vi "setup_MFLI.vi"(1 "Handle In":T1 {"Handle" format="0x%08x"; "Conn" format="0x%08x"}) -> (0 "Handle Out":T1 {"Handle" format="0x%08x"; "Conn" format="0x%08x"})   [LabVIEW 2019]
uses:
  Monitor Communication/zurich_lock_in/MFLIMonitor-Settings-Cluster.ctl
  Equipment/Zurich Instruments LabOne/Public/ziTypeHandle.ctl
  Instrument_Setup.vi
  Equipment/Zurich Instruments LabOne/Public/Configure/ziSetValueDouble.vi
  Equipment/Zurich Instruments LabOne/Zurich Instruments LabOne.lvlib
panel:
  out "MFLI-1-Settings":T2={"Adress"="DEV4756", "Osc 0 Freq"=0.0, "Osc 1 Freq"=0.0, "Osc 2 Freq"=0.0, "Osc 3 Freq"=0.0, "Demod 0 Osc"=0, "Demod 0 Harm"=1, "Demod 0 Phase"=0.0, "Demod 1 Osc"=0, "Demod 2 Osc"=0, "Demod 3 Osc"=0, "Demod 1 Harm"=1, "Demod 2 Harm"=1, "Demod 3 Harm"=1, "Demod 1 Phase"=0.0, "Demod 2 Phase"=0.0, "Demod 3 Phase"=0.0, "Input Demod 0"="", "Input Demod 1"="", "Input Demod 2"="", "Input Demod 3"="", "Demod 0 Order"=1, "Demod 0 TC"=0.0, "Demod 0 Sinc"=FALSE, "Demod 1 Order"=1, "Demod 2 Order"=1, "Demod 3 Order"=1, "Demod 1 TC"=0.0, "Demod 2 TC"=0.0, "Demod 3 TC"=0.0, "Demod 1 Sinc"=FALSE, "Demod 2 Sinc"=FALSE, "Demod 3 Sinc"=FALSE, "Demod 0 Enable"=FALSE, "Demod 0 Data Rate"=0.0, "Demod 1 Enable"=FALSE, "Demod 2 Enable"=FALSE, "Demod 3 Enable"=FALSE, "Demod 1 Data Rate"=0.0, "Demod 2 Data Rate"=0.0, "Demod 3 Data Rate"=0.0, "Ampl 0"=0.0, "Ampl 0 Enable"=FALSE, "Ampl 1"=0.0, "Ampl 2"=0.0, "Ampl 3"=0.0, "Ampl 1 Enable"=FALSE, "Ampl 2 Enable"=FALSE, "Ampl 3 Enable"=FALSE, "On"=FALSE, "50 Ohm"=FALSE, "Range (V)"=0.0, "Add"=FALSE, "Diff"=FALSE, "Auto-Range"=FALSE, "Offset (V)"=0.0, "Aux Out 0 Select"="", "Aux Out 0 Demod Num"=0.0, "Aux Out 0 Pre Offset"=0.0, "Aux Out 0 Scale"=0.0, "Aux Out 0 Offset"=0.0, "Aux Out 1 Select"="", "Aux Out 2 Select"="", "Aux Out 3 Select"="", "Aux Out 1 Pre Offset"=0.0, "Aux Out 2 Pre Offset"=0.0, "Aux Out 3 Pre Offset"=0.0, "Aux Out 1 Scale"=0.0, "Aux Out 2 Scale"=0.0, "Aux Out 3 Scale"=0.0, "Aux Out 1 Offset"=0.0, "Aux Out 2 Offset"=0.0, "Aux Out 3 Offset"=0.0, "Aux Out 1 Demod Num"=0.0, "Aux Out 2 Demod Num "=0.0, "Aux Out 3 Demod Num"=0.0, "Output Range (V)"=0.0} {"Aux Out 3 Demod Num" min=0.0 max=3.0 step=1.0; "Aux Out 2 Demod Num" min=0.0 max=3.0 step=1.0; "Aux Out 1 Demod Num" min=0.0 max=3.0 step=1.0; "Aux Out 0 Demod Num" min=0.0 max=3.0 step=1.0; "Demod 3 TC" min=0.0; "Demod 2 TC" min=0.0; "Demod 1 TC" min=0.0; "Demod 3 Order" min=1 max=8 step=1; "Demod 2 Order" min=1 max=8 step=1; "Demod 1 Order" min=1 max=8 step=1; "Demod 0 TC" min=0.0; "Demod 0 Order" min=1 max=8 step=1; "Demod 3 Phase" min=0.0 max=360.0; "Demod 2 Phase" min=0.0 max=360.0; "Demod 1 Phase" min=0.0 max=360.0; "Demod 3 Harm" min=1 max=1023 step=1; "Demod 2 Harm" min=1 max=1023 step=1; "Demod 1 Harm" min=1 max=1023 step=1; "Demod 3 Osc" min=0 max=3 step=1; "Demod 2 Osc" min=0 max=3 step=1; "Demod 1 Osc" min=0 max=3 step=1; "Demod 0 Phase" min=0.0 max=360.0; "Demod 0 Harm" min=1 max=1023 step=1; "Demod 0 Osc" min=0 max=3 step=1; "Osc 3 Freq" min=0.0 max=510000.0 format="%#_11g"; "Osc 2 Freq" min=0.0 max=510000.0 format="%#_11g"; "Osc 1 Freq" min=0.0 max=510000.0 format="%#_11g"; "Osc 0 Freq" min=0.0 max=510000.0 format="%#_11g"}
  # "Oscillators"
  # "Demodulators"
  # "Low-Pass Filter"
  # "Data Transfer"
  # "Output Amplitudes"
  # "Signal Outputs"
  # "Frequency (Hz)"
  # "Osc (#)"
  # "Harm (#)"
  # "Phase Offset (°)"
  # "Input"
  # "Order (#)"
  # "TC (s)"
  # "Sinc"
  # "Enabled"
  # "Rate (1/s)"
  # "Ampl (Vpk)"
  # "Enable"
  # "0"
  # "0"
  # "0"
  # "1"
  # "1"
  # "1"
  # "2"
  # "2"
  # "2"
  # "3"
  # "3"
  # "3"
  # "Output"
  # "Demod"
  # "Pre Offset"
  # "Scale"
  # "Offset"
  # "0"
  # "1"
  # "2"
  # "3"
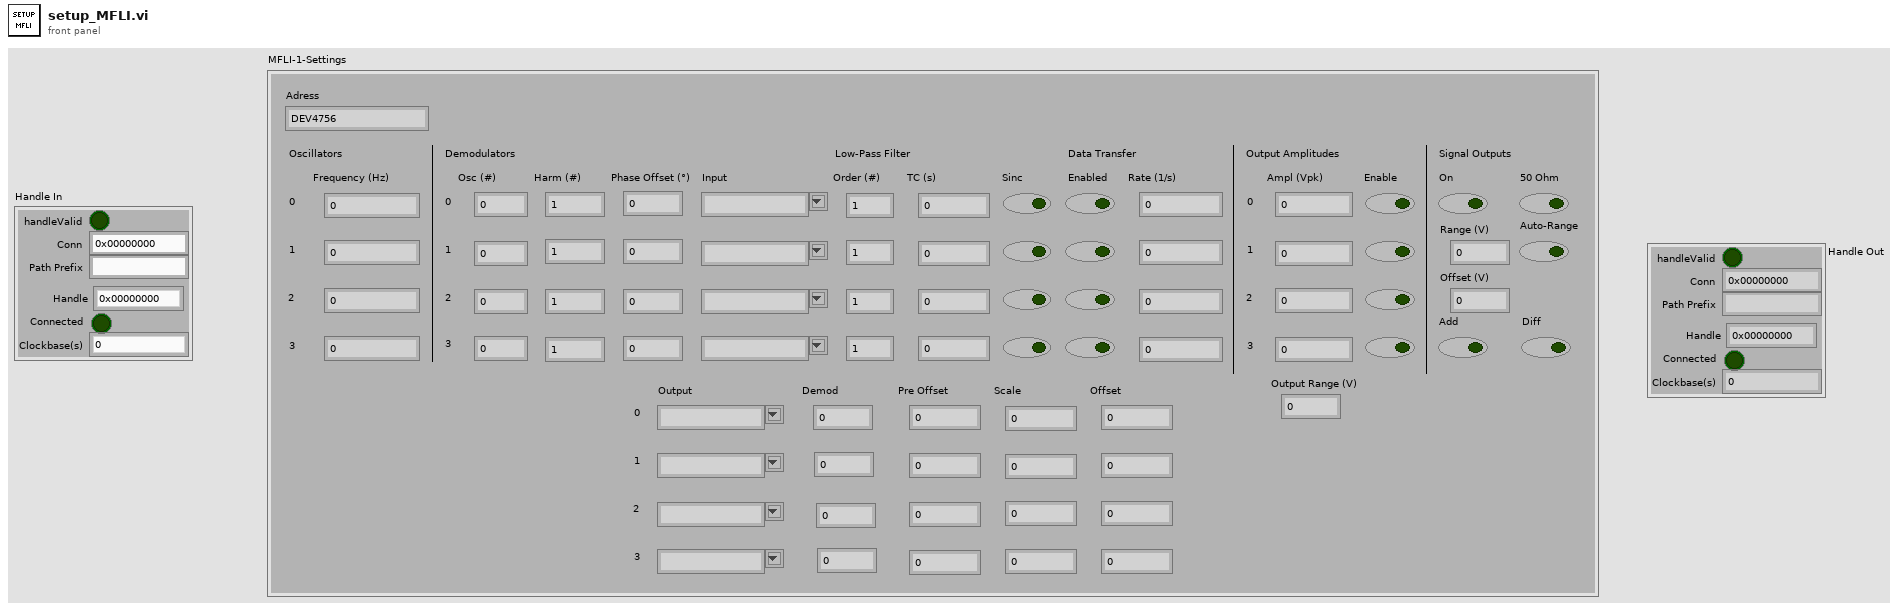
[diagram p1: front panel]
types:
  T1 = typedef "Zurich Instruments LabOne.lvlib/ziTypeHandle.ctl" = cluster{"handleValid":bool, "Conn":u64, "Path Prefix":string, "Handle":u64, "Connected":bool, "Clockbase(s)":dbl}
  T2 = typedef "MFLIMonitor-Settings-Cluster.ctl" = cluster{"Adress":string, "Osc 0 Freq":dbl, "Osc 1 Freq":dbl, "Osc 2 Freq":dbl, "Osc 3 Freq":dbl, "Demod 0 Osc":i8, "Demod 0 Harm":i16, "Demod 0 Phase":dbl, "Demod 1 Osc":i8, "Demod 2 Osc":i8, "Demod 3 Osc":i8, "Demod 1 Harm":i16, "Demod 2 Harm":i16, "Demod 3 Harm":i16, "Demod 1 Phase":dbl, "Demod 2 Phase":dbl, "Demod 3 Phase":dbl, "Input Demod 0":string, "Input Demod 1":string, "Input Demod 2":string, "Input Demod 3":string, "Demod 0 Order":i8, "Demod 0 TC":dbl, "Demod 0 Sinc":bool, "Demod 1 Order":i8, "Demod 2 Order":i8, "Demod 3 Order":i8, "Demod 1 TC":dbl, "Demod 2 TC":dbl, "Demod 3 TC":dbl, "Demod 1 Sinc":bool, "Demod 2 Sinc":bool, "Demod 3 Sinc":bool, "Demod 0 Enable":bool, "Demod 0 Data Rate":dbl, "Demod 1 Enable":bool, "Demod 2 Enable":bool, "Demod 3 Enable":bool, "Demod 1 Data Rate":dbl, "Demod 2 Data Rate":dbl, "Demod 3 Data Rate":dbl, "Ampl 0":dbl, "Ampl 0 Enable":bool, "Ampl 1":dbl, "Ampl 2":dbl, "Ampl 3":dbl, "Ampl 1 Enable":bool, "Ampl 2 Enable":bool, "Ampl 3 Enable":bool, "On":bool, "50 Ohm":bool, "Range (V)":dbl, "Add":bool, "Diff":bool, "Auto-Range":bool, "Offset (V)":dbl, "Aux Out 0 Select":string, "Aux Out 0 Demod Num":dbl, "Aux Out 0 Pre Offset":dbl, "Aux Out 0 Scale":dbl, "Aux Out 0 Offset":dbl, "Aux Out 1 Select":string, "Aux Out 2 Select":string, "Aux Out 3 Select":string, "Aux Out 1 Pre Offset":dbl, "Aux Out 2 Pre Offset":dbl, "Aux Out 3 Pre Offset":dbl, "Aux Out 1 Scale":dbl, "Aux Out 2 Scale":dbl, "Aux Out 3 Scale":dbl, "Aux Out 1 Offset":dbl, "Aux Out 2 Offset":dbl, "Aux Out 3 Offset":dbl, "Aux Out 1 Demod Num":dbl, "Aux Out 2 Demod Num ":dbl, "Aux Out 3 Demod Num":dbl, "Output Range (V)":dbl}
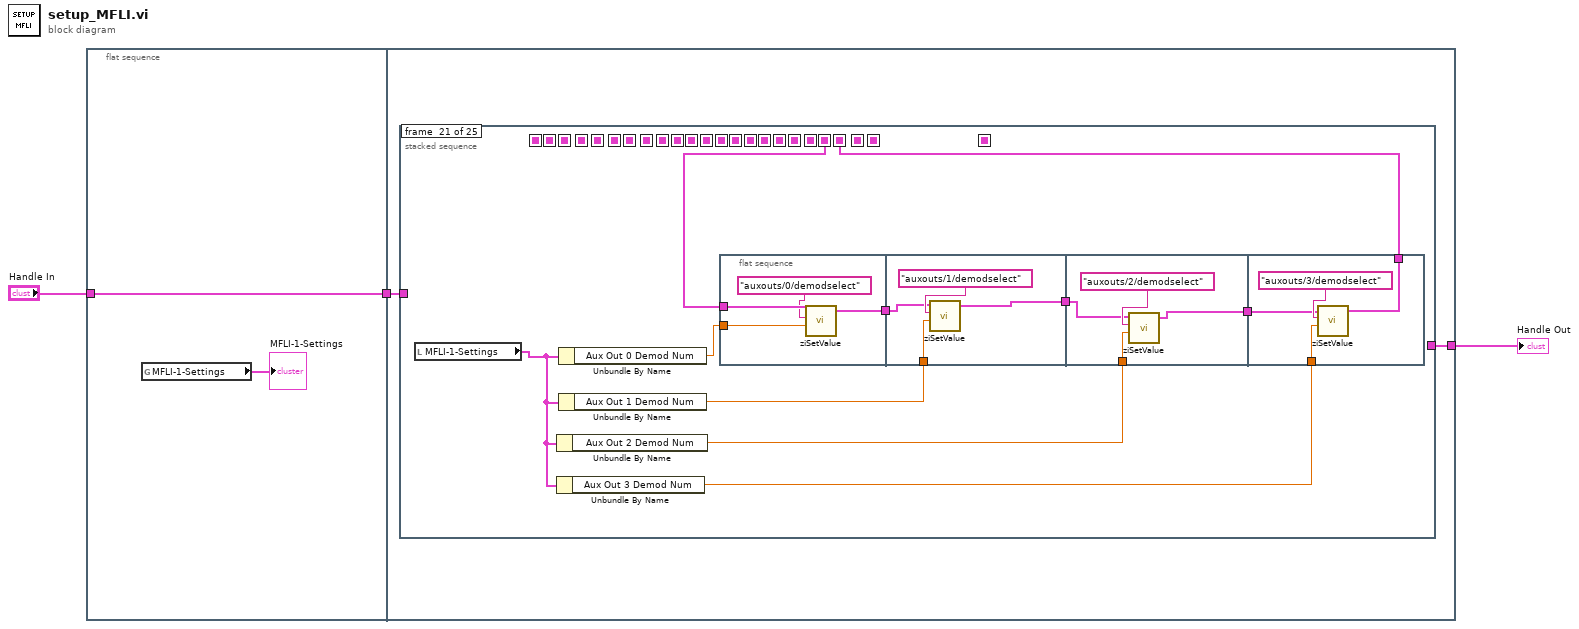
[diagram p0: block diagram]
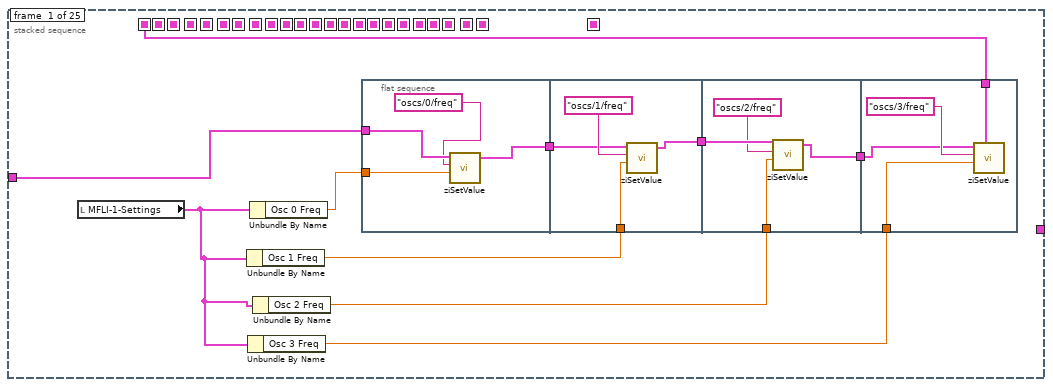
[diagram p2: hidden frame]
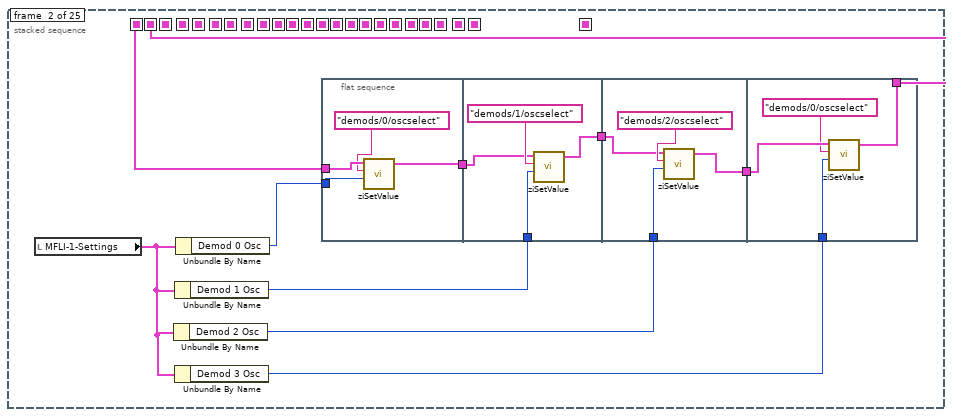
[diagram p3: hidden frame]
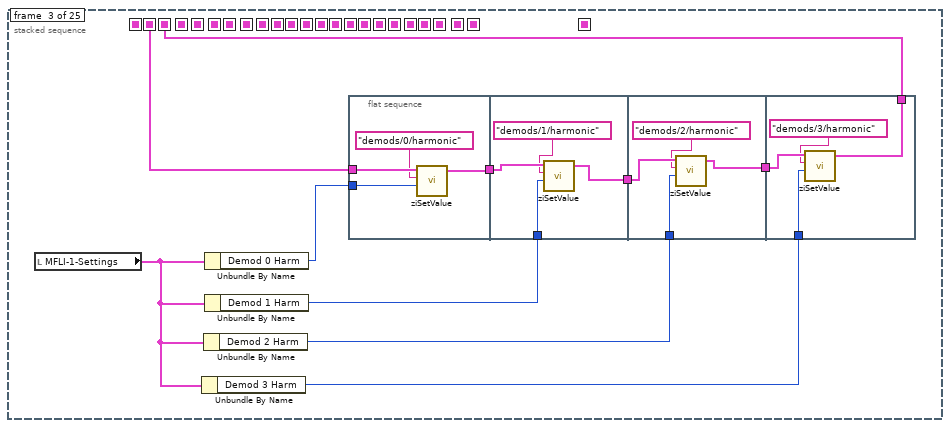
[diagram p4: hidden frame]
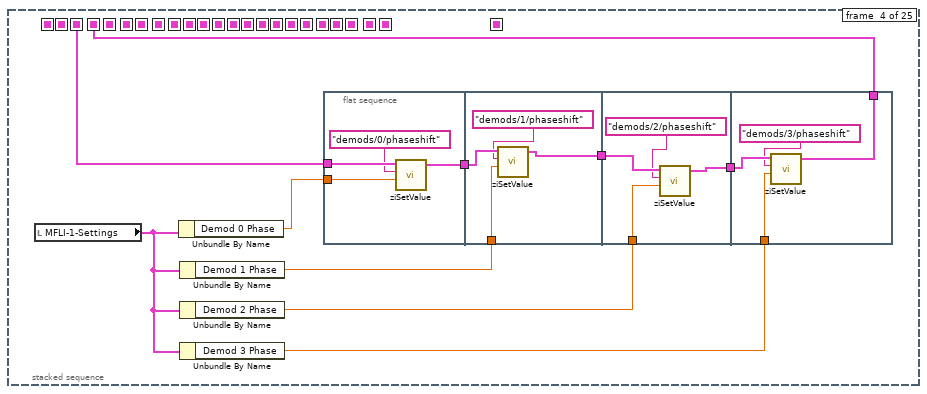
[diagram p5: hidden frame]
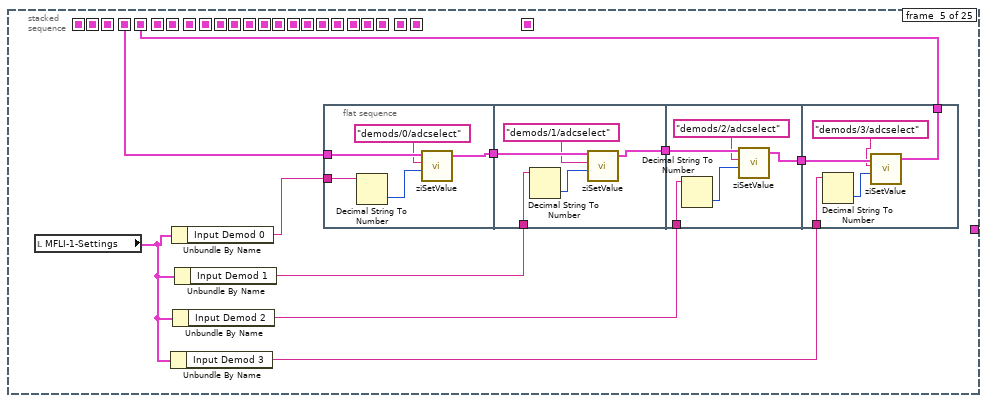
[diagram p6: hidden frame]
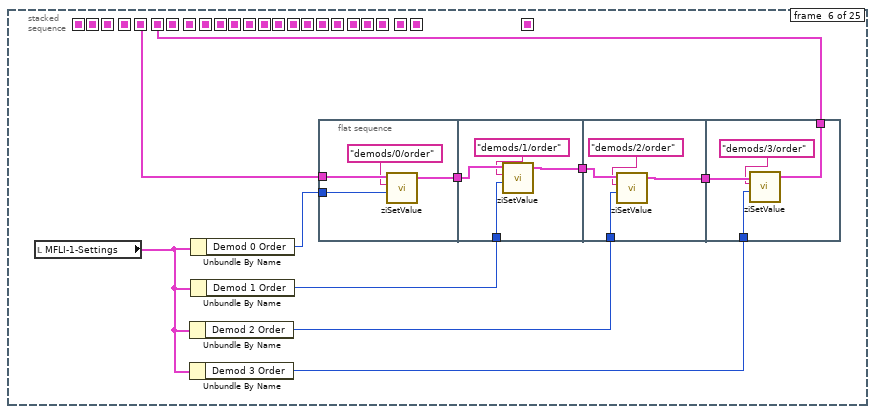
[diagram p7: hidden frame]
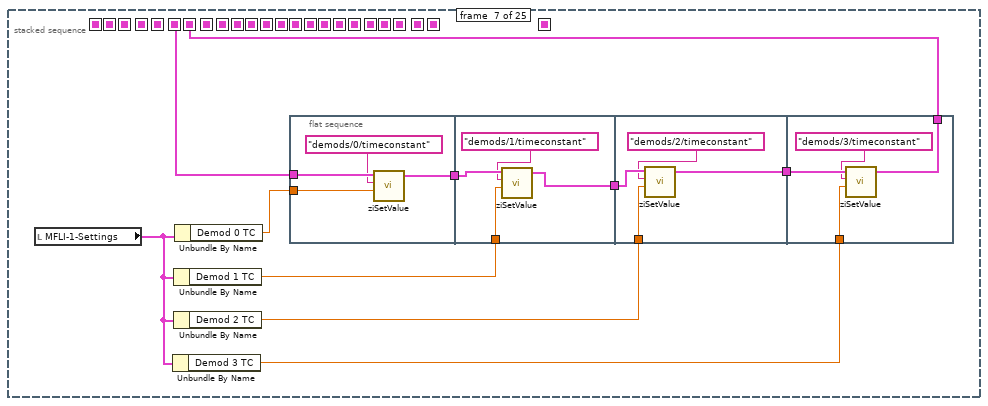
[diagram p8: hidden frame]
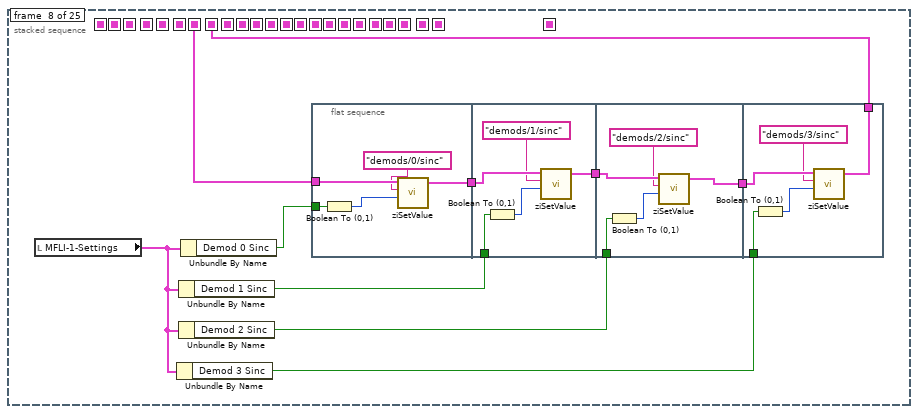
[diagram p9: hidden frame]
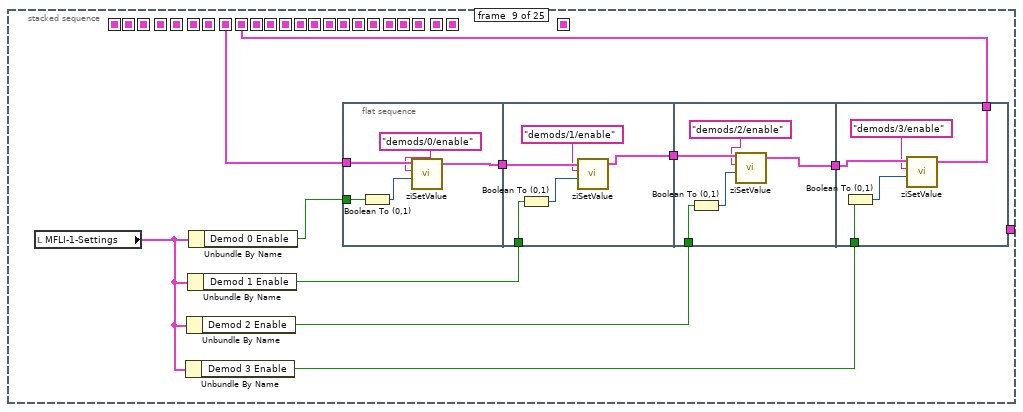
[diagram p10: hidden frame]
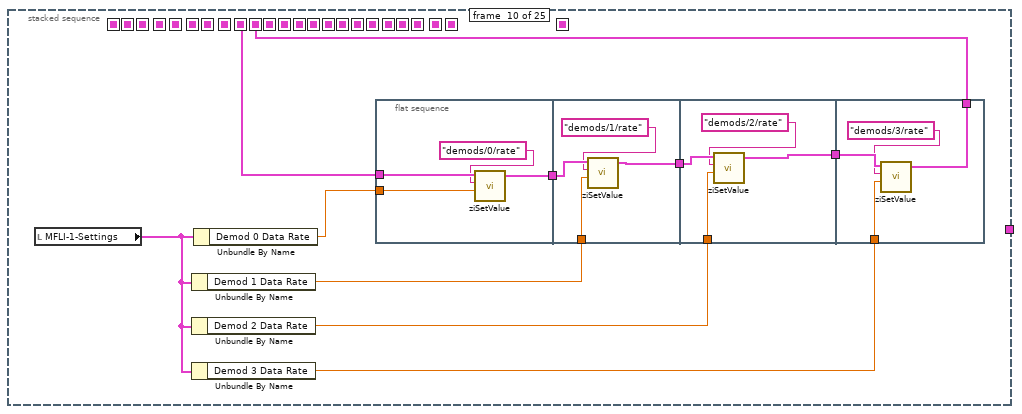
[diagram p11: hidden frame]
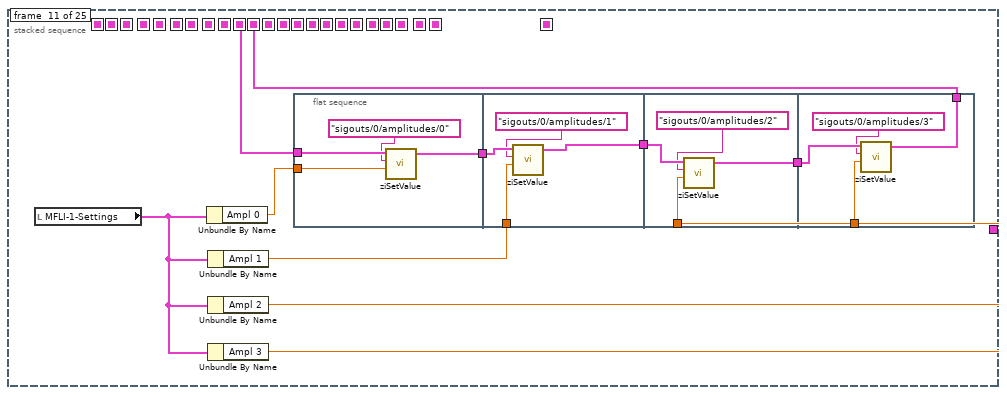
[diagram p12: hidden frame]
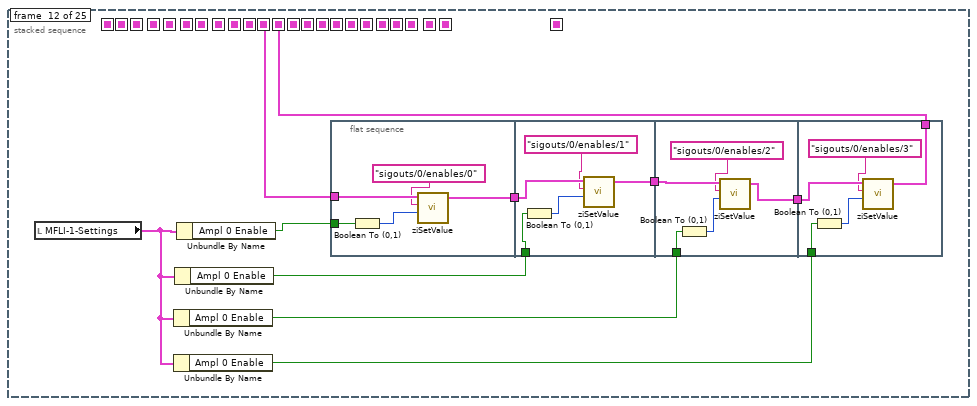
[diagram p13: hidden frame]
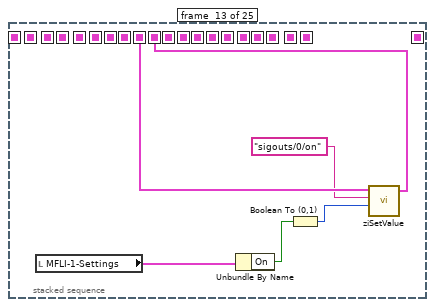
[diagram p14: hidden frame]
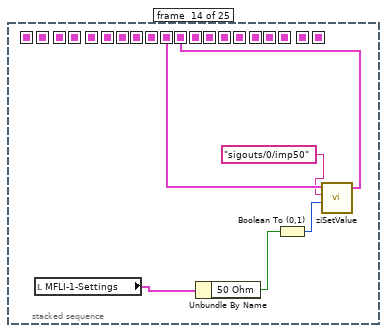
[diagram p15: hidden frame]
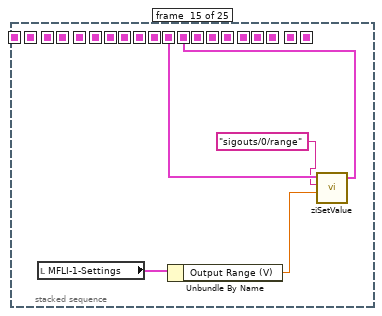
[diagram p16: hidden frame]
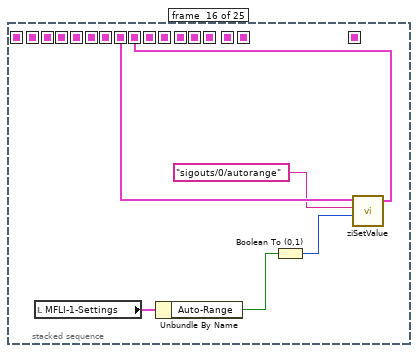
[diagram p17: hidden frame]
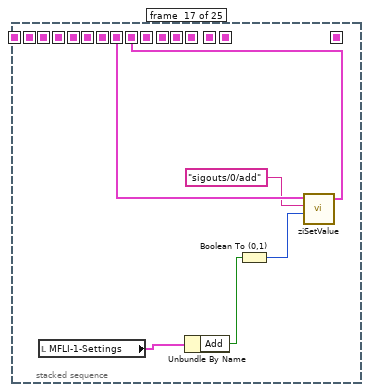
[diagram p18: hidden frame]
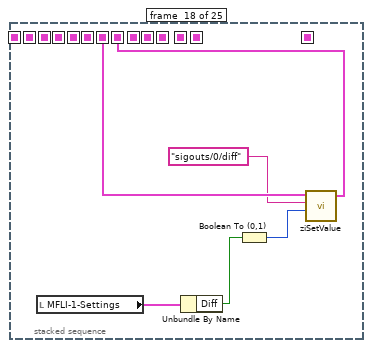
[diagram p19: hidden frame]
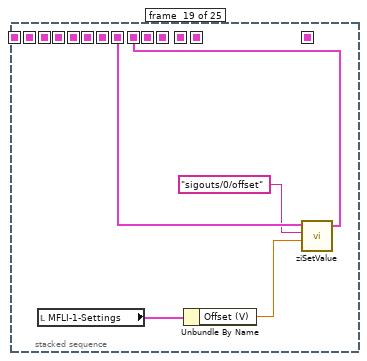
[diagram p20: hidden frame]
diagram:
  n1 = flat-sequence {
    tunnel: "Handle In" -> [w5]
    tunnel: [w5] -> w1
    tunnel: [w6] -> w2
    tunnel: w1 -> [w7]
    frame #0 {
      n2 = global read "Instrument_Setup.vi" "MFLI-1-Settings"() -> (→"MFLI-1-Settings":T2)
    }
    frame #1 {
      n3 = stacked-sequence {
        seq-local: [w8 _ _ _ _ _ _ _ _ _ _ _ _ _ _ _ _ _ _ _ _ _ _ _ _] -> [_ w43 _ _ _ _ _ _ _ _ _ _ _ _ _ _ _ _ _ _ _ _ _ _ _]
        seq-local: [_ w34 _ _ _ _ _ _ _ _ _ _ _ _ _ _ _ _ _ _ _ _ _ _ _] -> [_ _ w69 _ _ _ _ _ _ _ _ _ _ _ _ _ _ _ _ _ _ _ _ _ _]
        seq-local: [_ _ w60 _ _ _ _ _ _ _ _ _ _ _ _ _ _ _ _ _ _ _ _ _ _] -> [_ _ _ w95 _ _ _ _ _ _ _ _ _ _ _ _ _ _ _ _ _ _ _ _ _]
        seq-local: [_ _ _ w86 _ _ _ _ _ _ _ _ _ _ _ _ _ _ _ _ _ _ _ _ _] -> [_ _ _ _ w121 _ _ _ _ _ _ _ _ _ _ _ _ _ _ _ _ _ _ _ _]
        seq-local: [_ _ _ _ w112 _ _ _ _ _ _ _ _ _ _ _ _ _ _ _ _ _ _ _ _] -> [_ _ _ _ _ w151 _ _ _ _ _ _ _ _ _ _ _ _ _ _ _ _ _ _ _]
        seq-local: [_ _ _ _ _ w142 _ _ _ _ _ _ _ _ _ _ _ _ _ _ _ _ _ _ _] -> [_ _ _ _ _ _ w177 _ _ _ _ _ _ _ _ _ _ _ _ _ _ _ _ _ _]
        seq-local: [_ _ _ _ _ _ w168 _ _ _ _ _ _ _ _ _ _ _ _ _ _ _ _ _ _] -> [_ _ _ _ _ _ _ w203 _ _ _ _ _ _ _ _ _ _ _ _ _ _ _ _ _]
        seq-local: [_ _ _ _ _ _ _ w194 _ _ _ _ _ _ _ _ _ _ _ _ _ _ _ _ _] -> [_ _ _ _ _ _ _ _ w233 _ _ _ _ _ _ _ _ _ _ _ _ _ _ _ _]
        seq-local: [_ _ _ _ _ _ _ _ w224 _ _ _ _ _ _ _ _ _ _ _ _ _ _ _ _] -> [_ _ _ _ _ _ _ _ _ w263 _ _ _ _ _ _ _ _ _ _ _ _ _ _ _]
        seq-local: [_ _ _ _ _ _ _ _ _ w254 _ _ _ _ _ _ _ _ _ _ _ _ _ _ _] -> [_ _ _ _ _ _ _ _ _ _ w289 _ _ _ _ _ _ _ _ _ _ _ _ _ _]
        seq-local: [_ _ _ _ _ _ _ _ _ _ w280 _ _ _ _ _ _ _ _ _ _ _ _ _ _] -> [_ _ _ _ _ _ _ _ _ _ _ w315 _ _ _ _ _ _ _ _ _ _ _ _ _]
        seq-local: [_ _ _ _ _ _ _ _ _ _ _ w306 _ _ _ _ _ _ _ _ _ _ _ _ _] -> [_ _ _ _ _ _ _ _ _ _ _ _ w341 _ _ _ _ _ _ _ _ _ _ _ _]
        seq-local: [_ _ _ _ _ _ _ _ _ _ _ _ w339 _ _ _ _ _ _ _ _ _ _ _ _] -> [_ _ _ _ _ _ _ _ _ _ _ _ _ w347 _ _ _ _ _ _ _ _ _ _ _]
        seq-local: [_ _ _ _ _ _ _ _ _ _ _ _ _ w345 _ _ _ _ _ _ _ _ _ _ _] -> [_ _ _ _ _ _ _ _ _ _ _ _ _ _ w352 _ _ _ _ _ _ _ _ _ _]
        seq-local: [_ _ _ _ _ _ _ _ _ _ _ _ _ _ w350 _ _ _ _ _ _ _ _ _ _] -> [_ _ _ _ _ _ _ _ _ _ _ _ _ _ _ w357 _ _ _ _ _ _ _ _ _]
        seq-local: [_ _ _ _ _ _ _ _ _ _ _ _ _ _ _ w356 _ _ _ _ _ _ _ _ _] -> [_ _ _ _ _ _ _ _ _ _ _ _ _ _ _ _ w363 _ _ _ _ _ _ _ _]
        seq-local: [_ _ _ _ _ _ _ _ _ _ _ _ _ _ _ _ w362 _ _ _ _ _ _ _ _] -> [_ _ _ _ _ _ _ _ _ _ _ _ _ _ _ _ _ w370 _ _ _ _ _ _ _]
        seq-local: [_ _ _ _ _ _ _ _ _ _ _ _ _ _ _ _ _ w368 _ _ _ _ _ _ _] -> [_ _ _ _ _ _ _ _ _ _ _ _ _ _ _ _ _ _ w375 _ _ _ _ _ _]
        seq-local: [_ _ _ _ _ _ _ _ _ _ _ _ _ _ _ _ _ _ w373 _ _ _ _ _ _] -> [_ _ _ _ _ _ _ _ _ _ _ _ _ _ _ _ _ _ _ w385 _ _ _ _ _]
        seq-local: [_ _ _ _ _ _ _ _ _ _ _ _ _ _ _ _ _ _ _ w376 _ _ _ _ _] -> [_ _ _ _ _ _ _ _ _ _ _ _ _ _ _ _ _ _ _ _ w415 _ _ _ _]
        seq-local: [_ _ _ _ _ _ _ _ _ _ _ _ _ _ _ _ _ _ _ _ w406 _ _ _ _] -> [_ _ _ _ _ _ _ _ _ _ _ _ _ _ _ _ _ _ _ _ _ w441 _ _ _]
        seq-local: [_ _ _ _ _ _ _ _ _ _ _ _ _ _ _ _ _ _ _ _ _ w432 _ _ _] -> [_ _ _ _ _ _ _ _ _ _ _ _ _ _ _ _ _ _ _ _ _ _ w467 _ _]
        seq-local: [_ _ _ _ _ _ _ _ _ _ _ _ _ _ _ _ _ _ _ _ _ _ w458 _ _] -> [_ _ _ _ _ _ _ _ _ _ _ _ _ _ _ _ _ _ _ _ _ _ _ w493 _]
        seq-local: [_ _ _ _ _ _ _ _ _ _ _ _ _ _ _ _ _ _ _ _ _ _ _ w484 _] -> [_ _ _ _ _ _ _ _ _ _ _ _ _ _ _ _ _ _ _ _ _ _ _ _ w514]
        tunnel: w7 -> [w17 _ _ _ _ _ _ _ _ _ _ _ _ _ _ _ _ _ _ _ _ _ _ _ _]
        tunnel: [_ _ _ _ _ _ _ _ _ _ _ _ _ _ _ _ _ _ _ _ _ _ _ _ w512] -> w6
        frame #0 {
          n4 = local read "MFLI-1-Settings"() -> (w15:T2)
          n5 = Unbundle By Name(w15) -> ("Osc 1 Freq"=w13:dbl)
          n6 = Unbundle By Name(w15) -> ("Osc 3 Freq"=w9:dbl)
          n7 = Unbundle By Name(w15) -> ("Osc 0 Freq"=w16:dbl)
          n8 = Unbundle By Name(w15) -> ("Osc 2 Freq"=w11:dbl)
          n9 = flat-sequence {
            tunnel: w17 -> [w21]
            tunnel: w16 -> [w18]
            tunnel: [w20] -> w14
            tunnel: w14 -> [w23]
            tunnel: w13 -> [w25]
            tunnel: [w22] -> w12
            tunnel: w12 -> [w28]
            tunnel: w11 -> [w29]
            tunnel: [w27] -> w10
            tunnel: w10 -> [w31]
            tunnel: w9 -> [w33]
            tunnel: [w30] -> w8
            frame #0 {
              n10 = call-poly "ziSetValue.vi"("Value"=w18, "Path"="oscs/0/freq", "Handle In"=w21) -> ("Handle Out"=w20:T1)  [unwired: 2 in, 1 out]
            }
            frame #1 {
              n11 = call-poly "ziSetValue.vi"("Value"=w25, "Path"="oscs/1/freq", "Handle In"=w23) -> ("Handle Out"=w22:T1)  [unwired: 2 in, 1 out]
            }
            frame #2 {
              n12 = call-poly "ziSetValue.vi"("Value"=w29, "Path"="oscs/2/freq", "Handle In"=w28) -> ("Handle Out"=w27:T1)  [unwired: 2 in, 1 out]
            }
            frame #3 {
              n13 = call-poly "ziSetValue.vi"("Value"=w33, "Path"="oscs/3/freq", "Handle In"=w31) -> ("Handle Out"=w30:T1)  [unwired: 2 in, 1 out]
            }
          }
        }
        frame #1 {
          n14 = local read "MFLI-1-Settings"() -> (w42:T2)
          n15 = Unbundle By Name(w42) -> ("Demod 2 Osc"=w37:i8)
          n16 = Unbundle By Name(w42) -> ("Demod 1 Osc"=w39:i8)
          n17 = Unbundle By Name(w42) -> ("Demod 3 Osc"=w35:i8)
          n18 = Unbundle By Name(w42) -> ("Demod 0 Osc"=w41:i8)
          n19 = flat-sequence {
            tunnel: w43 -> [w47]
            tunnel: w41 -> [w44]
            tunnel: [w46] -> w40
            tunnel: w40 -> [w49]
            tunnel: w39 -> [w51]
            tunnel: [w48] -> w38
            tunnel: w38 -> [w53]
            tunnel: w37 -> [w55]
            tunnel: [w52] -> w36
            tunnel: w36 -> [w58]
            tunnel: w35 -> [w59]
            tunnel: [w57] -> w34
            frame #0 {
              n20 = call-poly "ziSetValue.vi"("Value"=w44, "Path"="demods/0/oscselect", "Handle In"=w47) -> ("Handle Out"=w46:T1)  [unwired: 2 in, 1 out]
            }
            frame #1 {
              n21 = call-poly "ziSetValue.vi"("Value"=w51, "Path"="demods/1/oscselect", "Handle In"=w49) -> ("Handle Out"=w48:T1)  [unwired: 2 in, 1 out]
            }
            frame #2 {
              n22 = call-poly "ziSetValue.vi"("Value"=w55, "Path"="demods/2/oscselect", "Handle In"=w53) -> ("Handle Out"=w52:T1)  [unwired: 2 in, 1 out]
            }
            frame #3 {
              n23 = call-poly "ziSetValue.vi"("Value"=w59, "Path"="demods/0/oscselect", "Handle In"=w58) -> ("Handle Out"=w57:T1)  [unwired: 2 in, 1 out]
            }
          }
        }
        frame #2 {
          n24 = local read "MFLI-1-Settings"() -> (w68:T2)
          n25 = Unbundle By Name(w68) -> ("Demod 3 Harm"=w61:i16)
          n26 = Unbundle By Name(w68) -> ("Demod 2 Harm"=w63:i16)
          n27 = Unbundle By Name(w68) -> ("Demod 0 Harm"=w67:i16)
          n28 = Unbundle By Name(w68) -> ("Demod 1 Harm"=w65:i16)
          n29 = flat-sequence {
            tunnel: w69 -> [w73]
            tunnel: w67 -> [w70]
            tunnel: [w72] -> w66
            tunnel: w66 -> [w76]
            tunnel: w65 -> [w77]
            tunnel: [w75] -> w64
            tunnel: w64 -> [w80]
            tunnel: w63 -> [w81]
            tunnel: [w79] -> w62
            tunnel: w62 -> [w84]
            tunnel: w61 -> [w85]
            tunnel: [w83] -> w60
            frame #0 {
              n30 = call-poly "ziSetValue.vi"("Value"=w70, "Path"="demods/0/harmonic", "Handle In"=w73) -> ("Handle Out"=w72:T1)  [unwired: 2 in, 1 out]
            }
            frame #1 {
              n31 = call-poly "ziSetValue.vi"("Value"=w77, "Path"="demods/1/harmonic", "Handle In"=w76) -> ("Handle Out"=w75:T1)  [unwired: 2 in, 1 out]
            }
            frame #2 {
              n32 = call-poly "ziSetValue.vi"("Value"=w81, "Path"="demods/2/harmonic", "Handle In"=w80) -> ("Handle Out"=w79:T1)  [unwired: 2 in, 1 out]
            }
            frame #3 {
              n33 = call-poly "ziSetValue.vi"("Value"=w85, "Path"="demods/3/harmonic", "Handle In"=w84) -> ("Handle Out"=w83:T1)  [unwired: 2 in, 1 out]
            }
          }
        }
        frame #3 {
          n34 = local read "MFLI-1-Settings"() -> (w94:T2)
          n35 = Unbundle By Name(w94) -> ("Demod 0 Phase"=w93:dbl)
          n36 = Unbundle By Name(w94) -> ("Demod 1 Phase"=w91:dbl)
          n37 = Unbundle By Name(w94) -> ("Demod 2 Phase"=w89:dbl)
          n38 = Unbundle By Name(w94) -> ("Demod 3 Phase"=w87:dbl)
          n39 = flat-sequence {
            tunnel: w95 -> [w99]
            tunnel: w93 -> [w96]
            tunnel: [w98] -> w92
            tunnel: w92 -> [w102]
            tunnel: w91 -> [w103]
            tunnel: [w101] -> w90
            tunnel: w90 -> [w106]
            tunnel: w89 -> [w107]
            tunnel: [w105] -> w88
            tunnel: w88 -> [w110]
            tunnel: w87 -> [w111]
            tunnel: [w109] -> w86
            frame #0 {
              n40 = call-poly "ziSetValue.vi"("Value"=w96, "Path"="demods/0/phaseshift", "Handle In"=w99) -> ("Handle Out"=w98:T1)  [unwired: 2 in, 1 out]
            }
            frame #1 {
              n41 = call-poly "ziSetValue.vi"("Value"=w103, "Path"="demods/1/phaseshift", "Handle In"=w102) -> ("Handle Out"=w101:T1)  [unwired: 2 in, 1 out]
            }
            frame #2 {
              n42 = call-poly "ziSetValue.vi"("Value"=w107, "Path"="demods/2/phaseshift", "Handle In"=w106) -> ("Handle Out"=w105:T1)  [unwired: 2 in, 1 out]
            }
            frame #3 {
              n43 = call-poly "ziSetValue.vi"("Value"=w111, "Path"="demods/3/phaseshift", "Handle In"=w110) -> ("Handle Out"=w109:T1)  [unwired: 2 in, 1 out]
            }
          }
        }
        frame #4 {
          n44 = local read "MFLI-1-Settings"() -> (w120:T2)
          n45 = Unbundle By Name(w120) -> ("Input Demod 3"=w113:string)
          n46 = Unbundle By Name(w120) -> ("Input Demod 0"=w119:string)
          n47 = Unbundle By Name(w120) -> ("Input Demod 2"=w115:string)
          n48 = Unbundle By Name(w120) -> ("Input Demod 1"=w117:string)
          n49 = flat-sequence {
            tunnel: w121 -> [w126]
            tunnel: w119 -> [w122]
            tunnel: [w125] -> w118
            tunnel: w118 -> [w129]
            tunnel: w117 -> [w131]
            tunnel: [w128] -> w116
            tunnel: w116 -> [w134]
            tunnel: w115 -> [w136]
            tunnel: [w133] -> w114
            tunnel: w114 -> [w139]
            tunnel: w113 -> [w141]
            tunnel: [w138] -> w112
            frame #0 {
              n50 = Decimal String To Number(string=w122) -> (number=w123:i32)  [unwired: 2 in, 1 out]
              n51 = call-poly "ziSetValue.vi"("Value"=w123, "Path"="demods/0/adcselect", "Handle In"=w126) -> ("Handle Out"=w125:T1)  [unwired: 2 in, 1 out]
            }
            frame #1 {
              n52 = Decimal String To Number(string=w131) -> (number=w130:i32)  [unwired: 2 in, 1 out]
              n53 = call-poly "ziSetValue.vi"("Value"=w130, "Path"="demods/1/adcselect", "Handle In"=w129) -> ("Handle Out"=w128:T1)  [unwired: 2 in, 1 out]
            }
            frame #2 {
              n54 = Decimal String To Number(string=w136) -> (number=w135:i32)  [unwired: 2 in, 1 out]
              n55 = call-poly "ziSetValue.vi"("Value"=w135, "Path"="demods/2/adcselect", "Handle In"=w134) -> ("Handle Out"=w133:T1)  [unwired: 2 in, 1 out]
            }
            frame #3 {
              n56 = Decimal String To Number(string=w141) -> (number=w140:i32)  [unwired: 2 in, 1 out]
              n57 = call-poly "ziSetValue.vi"("Value"=w140, "Path"="demods/3/adcselect", "Handle In"=w139) -> ("Handle Out"=w138:T1)  [unwired: 2 in, 1 out]
            }
          }
        }
        frame #5 {
          n58 = local read "MFLI-1-Settings"() -> (w150:T2)
          n59 = Unbundle By Name(w150) -> ("Demod 2 Order"=w145:i8)
          n60 = Unbundle By Name(w150) -> ("Demod 3 Order"=w143:i8)
          n61 = Unbundle By Name(w150) -> ("Demod 0 Order"=w149:i8)
          n62 = Unbundle By Name(w150) -> ("Demod 1 Order"=w147:i8)
          n63 = flat-sequence {
            tunnel: w151 -> [w155]
            tunnel: w149 -> [w152]
            tunnel: [w154] -> w148
            tunnel: w148 -> [w158]
            tunnel: w147 -> [w159]
            tunnel: [w157] -> w146
            tunnel: w146 -> [w162]
            tunnel: w145 -> [w163]
            tunnel: [w161] -> w144
            tunnel: w144 -> [w166]
            tunnel: w143 -> [w167]
            tunnel: [w165] -> w142
            frame #0 {
              n64 = call-poly "ziSetValue.vi"("Value"=w152, "Path"="demods/0/order", "Handle In"=w155) -> ("Handle Out"=w154:T1)  [unwired: 2 in, 1 out]
            }
            frame #1 {
              n65 = call-poly "ziSetValue.vi"("Value"=w159, "Path"="demods/1/order", "Handle In"=w158) -> ("Handle Out"=w157:T1)  [unwired: 2 in, 1 out]
            }
            frame #2 {
              n66 = call-poly "ziSetValue.vi"("Value"=w163, "Path"="demods/2/order", "Handle In"=w162) -> ("Handle Out"=w161:T1)  [unwired: 2 in, 1 out]
            }
            frame #3 {
              n67 = call-poly "ziSetValue.vi"("Value"=w167, "Path"="demods/3/order", "Handle In"=w166) -> ("Handle Out"=w165:T1)  [unwired: 2 in, 1 out]
            }
          }
        }
        frame #6 {
          n68 = local read "MFLI-1-Settings"() -> (w176:T2)
          n69 = Unbundle By Name(w176) -> ("Demod 3 TC"=w169:dbl)
          n70 = Unbundle By Name(w176) -> ("Demod 1 TC"=w173:dbl)
          n71 = Unbundle By Name(w176) -> ("Demod 2 TC"=w171:dbl)
          n72 = Unbundle By Name(w176) -> ("Demod 0 TC"=w175:dbl)
          n73 = flat-sequence {
            tunnel: w177 -> [w181]
            tunnel: w175 -> [w178]
            tunnel: [w180] -> w174
            tunnel: w174 -> [w184]
            tunnel: w173 -> [w185]
            tunnel: [w183] -> w172
            tunnel: w172 -> [w188]
            tunnel: w171 -> [w189]
            tunnel: [w187] -> w170
            tunnel: w170 -> [w192]
            tunnel: w169 -> [w193]
            tunnel: [w191] -> w168
            frame #0 {
              n74 = call-poly "ziSetValue.vi"("Value"=w178, "Path"="demods/0/timeconstant", "Handle In"=w181) -> ("Handle Out"=w180:T1)  [unwired: 2 in, 1 out]
            }
            frame #1 {
              n75 = call-poly "ziSetValue.vi"("Value"=w185, "Path"="demods/1/timeconstant", "Handle In"=w184) -> ("Handle Out"=w183:T1)  [unwired: 2 in, 1 out]
            }
            frame #2 {
              n76 = call-poly "ziSetValue.vi"("Value"=w189, "Path"="demods/2/timeconstant", "Handle In"=w188) -> ("Handle Out"=w187:T1)  [unwired: 2 in, 1 out]
            }
            frame #3 {
              n77 = call-poly "ziSetValue.vi"("Value"=w193, "Path"="demods/3/timeconstant", "Handle In"=w192) -> ("Handle Out"=w191:T1)  [unwired: 2 in, 1 out]
            }
          }
        }
        frame #7 {
          n78 = local read "MFLI-1-Settings"() -> (w202:T2)
          n79 = Unbundle By Name(w202) -> ("Demod 3 Sinc"=w195:bool)
          n80 = Unbundle By Name(w202) -> ("Demod 1 Sinc"=w199:bool)
          n81 = Unbundle By Name(w202) -> ("Demod 2 Sinc"=w197:bool)
          n82 = Unbundle By Name(w202) -> ("Demod 0 Sinc"=w201:bool)
          n83 = flat-sequence {
            tunnel: w203 -> [w208]
            tunnel: w201 -> [w204]
            tunnel: [w207] -> w200
            tunnel: w200 -> [w211]
            tunnel: w199 -> [w213]
            tunnel: [w210] -> w198
            tunnel: w198 -> [w216]
            tunnel: w197 -> [w218]
            tunnel: [w215] -> w196
            tunnel: w196 -> [w221]
            tunnel: w195 -> [w223]
            tunnel: [w220] -> w194
            frame #0 {
              n84 = Boolean To (0,1)(Boolean=w204) -> (0, 1=w205:i16)
              n85 = call-poly "ziSetValue.vi"("Value"=w205, "Path"="demods/0/sinc", "Handle In"=w208) -> ("Handle Out"=w207:T1)  [unwired: 2 in, 1 out]
            }
            frame #1 {
              n86 = Boolean To (0,1)(Boolean=w213) -> (0, 1=w212:i16)
              n87 = call-poly "ziSetValue.vi"("Value"=w212, "Path"="demods/1/sinc", "Handle In"=w211) -> ("Handle Out"=w210:T1)  [unwired: 2 in, 1 out]
            }
            frame #2 {
              n88 = Boolean To (0,1)(Boolean=w218) -> (0, 1=w217:i16)
              n89 = call-poly "ziSetValue.vi"("Value"=w217, "Path"="demods/2/sinc", "Handle In"=w216) -> ("Handle Out"=w215:T1)  [unwired: 2 in, 1 out]
            }
            frame #3 {
              n90 = Boolean To (0,1)(Boolean=w223) -> (0, 1=w222:i16)
              n91 = call-poly "ziSetValue.vi"("Value"=w222, "Path"="demods/3/sinc", "Handle In"=w221) -> ("Handle Out"=w220:T1)  [unwired: 2 in, 1 out]
            }
          }
        }
        frame #8 {
          n92 = local read "MFLI-1-Settings"() -> (w232:T2)
          n93 = Unbundle By Name(w232) -> ("Demod 3 Enable"=w225:bool)
          n94 = Unbundle By Name(w232) -> ("Demod 2 Enable"=w227:bool)
          n95 = Unbundle By Name(w232) -> ("Demod 1 Enable"=w229:bool)
          n96 = Unbundle By Name(w232) -> ("Demod 0 Enable"=w231:bool)
          n97 = flat-sequence {
            tunnel: w233 -> [w238]
            tunnel: w231 -> [w234]
            tunnel: [w237] -> w230
            tunnel: w230 -> [w241]
            tunnel: w229 -> [w243]
            tunnel: [w240] -> w228
            tunnel: w228 -> [w246]
            tunnel: w227 -> [w248]
            tunnel: [w245] -> w226
            tunnel: w226 -> [w251]
            tunnel: w225 -> [w253]
            tunnel: [w250] -> w224
            frame #0 {
              n98 = Boolean To (0,1)(Boolean=w234) -> (0, 1=w235:i16)
              n99 = call-poly "ziSetValue.vi"("Value"=w235, "Path"="demods/0/enable", "Handle In"=w238) -> ("Handle Out"=w237:T1)  [unwired: 2 in, 1 out]
            }
            frame #1 {
              n100 = Boolean To (0,1)(Boolean=w243) -> (0, 1=w242:i16)
              n101 = call-poly "ziSetValue.vi"("Value"=w242, "Path"="demods/1/enable", "Handle In"=w241) -> ("Handle Out"=w240:T1)  [unwired: 2 in, 1 out]
            }
            frame #2 {
              n102 = Boolean To (0,1)(Boolean=w248) -> (0, 1=w247:i16)
              n103 = call-poly "ziSetValue.vi"("Value"=w247, "Path"="demods/2/enable", "Handle In"=w246) -> ("Handle Out"=w245:T1)  [unwired: 2 in, 1 out]
            }
            frame #3 {
              n104 = Boolean To (0,1)(Boolean=w253) -> (0, 1=w252:i16)
              n105 = call-poly "ziSetValue.vi"("Value"=w252, "Path"="demods/3/enable", "Handle In"=w251) -> ("Handle Out"=w250:T1)  [unwired: 2 in, 1 out]
            }
          }
        }
        frame #9 {
          n106 = local read "MFLI-1-Settings"() -> (w262:T2)
          n107 = Unbundle By Name(w262) -> ("Demod 1 Data Rate"=w259:dbl)
          n108 = Unbundle By Name(w262) -> ("Demod 2 Data Rate"=w257:dbl)
          n109 = Unbundle By Name(w262) -> ("Demod 3 Data Rate"=w255:dbl)
          n110 = Unbundle By Name(w262) -> ("Demod 0 Data Rate"=w261:dbl)
          n111 = flat-sequence {
            tunnel: w263 -> [w267]
            tunnel: w261 -> [w264]
            tunnel: [w266] -> w260
            tunnel: w260 -> [w270]
            tunnel: w259 -> [w271]
            tunnel: [w269] -> w258
            tunnel: w258 -> [w274]
            tunnel: w257 -> [w275]
            tunnel: [w273] -> w256
            tunnel: w256 -> [w278]
            tunnel: w255 -> [w279]
            tunnel: [w277] -> w254
            frame #0 {
              n112 = call-poly "ziSetValue.vi"("Value"=w264, "Path"="demods/0/rate", "Handle In"=w267) -> ("Handle Out"=w266:T1)  [unwired: 2 in, 1 out]
            }
            frame #1 {
              n113 = call-poly "ziSetValue.vi"("Value"=w271, "Path"="demods/1/rate", "Handle In"=w270) -> ("Handle Out"=w269:T1)  [unwired: 2 in, 1 out]
            }
            frame #2 {
              n114 = call-poly "ziSetValue.vi"("Value"=w275, "Path"="demods/2/rate", "Handle In"=w274) -> ("Handle Out"=w273:T1)  [unwired: 2 in, 1 out]
            }
            frame #3 {
              n115 = call-poly "ziSetValue.vi"("Value"=w279, "Path"="demods/3/rate", "Handle In"=w278) -> ("Handle Out"=w277:T1)  [unwired: 2 in, 1 out]
            }
          }
        }
        frame #10 {
          n116 = local read "MFLI-1-Settings"() -> (w288:T2)
          n117 = Unbundle By Name(w288) -> ("Ampl 0"=w287:dbl)
          n118 = Unbundle By Name(w288) -> ("Ampl 1"=w285:dbl)
          n119 = Unbundle By Name(w288) -> ("Ampl 2"=w283:dbl)
          n120 = Unbundle By Name(w288) -> ("Ampl 3"=w281:dbl)
          n121 = flat-sequence {
            tunnel: w289 -> [w293]
            tunnel: w287 -> [w290]
            tunnel: [w292] -> w286
            tunnel: w286 -> [w296]
            tunnel: w285 -> [w297]
            tunnel: [w295] -> w284
            tunnel: w284 -> [w300]
            tunnel: w283 -> [w301]
            tunnel: [w299] -> w282
            tunnel: w282 -> [w304]
            tunnel: w281 -> [w305]
            tunnel: [w303] -> w280
            frame #0 {
              n122 = call-poly "ziSetValue.vi"("Value"=w290, "Path"="sigouts/0/amplitudes/0", "Handle In"=w293) -> ("Handle Out"=w292:T1)  [unwired: 2 in, 1 out]
            }
            frame #1 {
              n123 = call-poly "ziSetValue.vi"("Value"=w297, "Path"="sigouts/0/amplitudes/1", "Handle In"=w296) -> ("Handle Out"=w295:T1)  [unwired: 2 in, 1 out]
            }
            frame #2 {
              n124 = call-poly "ziSetValue.vi"("Value"=w301, "Path"="sigouts/0/amplitudes/2", "Handle In"=w300) -> ("Handle Out"=w299:T1)  [unwired: 2 in, 1 out]
            }
            frame #3 {
              n125 = call-poly "ziSetValue.vi"("Value"=w305, "Path"="sigouts/0/amplitudes/3", "Handle In"=w304) -> ("Handle Out"=w303:T1)  [unwired: 2 in, 1 out]
            }
          }
        }
        frame #11 {
          n126 = local read "MFLI-1-Settings"() -> (w314:T2)
          n127 = Unbundle By Name(w314) -> ("Ampl 0 Enable"=w309:bool)
          n128 = Unbundle By Name(w314) -> ("Ampl 0 Enable"=w307:bool)
          n129 = Unbundle By Name(w314) -> ("Ampl 0 Enable"=w311:bool)
          n130 = Unbundle By Name(w314) -> ("Ampl 0 Enable"=w313:bool)
          n131 = flat-sequence {
            tunnel: w315 -> [w320]
            tunnel: w313 -> [w316]
            tunnel: [w319] -> w312
            tunnel: w312 -> [w323]
            tunnel: w311 -> [w325]
            tunnel: [w322] -> w310
            tunnel: w310 -> [w328]
            tunnel: w309 -> [w330]
            tunnel: [w327] -> w308
            tunnel: w308 -> [w333]
            tunnel: w307 -> [w335]
            tunnel: [w332] -> w306
            frame #0 {
              n132 = Boolean To (0,1)(Boolean=w316) -> (0, 1=w317:i16)
              n133 = call-poly "ziSetValue.vi"("Value"=w317, "Path"="sigouts/0/enables/0", "Handle In"=w320) -> ("Handle Out"=w319:T1)  [unwired: 2 in, 1 out]
            }
            frame #1 {
              n134 = Boolean To (0,1)(Boolean=w325) -> (0, 1=w324:i16)
              n135 = call-poly "ziSetValue.vi"("Value"=w324, "Path"="sigouts/0/enables/1", "Handle In"=w323) -> ("Handle Out"=w322:T1)  [unwired: 2 in, 1 out]
            }
            frame #2 {
              n136 = Boolean To (0,1)(Boolean=w330) -> (0, 1=w329:i16)
              n137 = call-poly "ziSetValue.vi"("Value"=w329, "Path"="sigouts/0/enables/2", "Handle In"=w328) -> ("Handle Out"=w327:T1)  [unwired: 2 in, 1 out]
            }
            frame #3 {
              n138 = Boolean To (0,1)(Boolean=w335) -> (0, 1=w334:i16)
              n139 = call-poly "ziSetValue.vi"("Value"=w334, "Path"="sigouts/0/enables/3", "Handle In"=w333) -> ("Handle Out"=w332:T1)  [unwired: 2 in, 1 out]
            }
          }
        }
        frame #12 {
          n140 = local read "MFLI-1-Settings"() -> (w340:T2)
          n141 = Unbundle By Name(w340) -> ("On"=w336:bool)
          n142 = Boolean To (0,1)(Boolean=w336) -> (0, 1=w337:i16)
          n143 = call-poly "ziSetValue.vi"("Value"=w337, "Path"="sigouts/0/on", "Handle In"=w341) -> ("Handle Out"=w339:T1)  [unwired: 2 in, 1 out]
        }
        frame #13 {
          n144 = local read "MFLI-1-Settings"() -> (w346:T2)
          n145 = Unbundle By Name(w346) -> ("50 Ohm"=w342:bool)
          n146 = Boolean To (0,1)(Boolean=w342) -> (0, 1=w343:i16)
          n147 = call-poly "ziSetValue.vi"("Value"=w343, "Path"="sigouts/0/imp50", "Handle In"=w347) -> ("Handle Out"=w345:T1)  [unwired: 2 in, 1 out]
        }
        frame #14 {
          n148 = local read "MFLI-1-Settings"() -> (w351:T2)
          n149 = Unbundle By Name(w351) -> ("Output Range (V)"=w348:dbl)
          n150 = call-poly "ziSetValue.vi"("Value"=w348, "Path"="sigouts/0/range", "Handle In"=w352) -> ("Handle Out"=w350:T1)  [unwired: 2 in, 1 out]
        }
        frame #15 {
          n151 = local read "MFLI-1-Settings"() -> (w358:T2)
          n152 = Unbundle By Name(w358) -> ("Auto-Range"=w353:bool)
          n153 = Boolean To (0,1)(Boolean=w353) -> (0, 1=w355:i16)
          n154 = call-poly "ziSetValue.vi"("Value"=w355, "Path"="sigouts/0/autorange", "Handle In"=w357) -> ("Handle Out"=w356:T1)  [unwired: 2 in, 1 out]
        }
        frame #16 {
          n155 = local read "MFLI-1-Settings"() -> (w364:T2)
          n156 = Unbundle By Name(w364) -> ("Add"=w359:bool)
          n157 = Boolean To (0,1)(Boolean=w359) -> (0, 1=w361:i16)
          n158 = call-poly "ziSetValue.vi"("Value"=w361, "Path"="sigouts/0/add", "Handle In"=w363) -> ("Handle Out"=w362:T1)  [unwired: 2 in, 1 out]
        }
        frame #17 {
          n159 = local read "MFLI-1-Settings"() -> (w369:T2)
          n160 = Unbundle By Name(w369) -> ("Diff"=w365:bool)
          n161 = Boolean To (0,1)(Boolean=w365) -> (0, 1=w366:i16)
          n162 = call-poly "ziSetValue.vi"("Value"=w366, "Path"="sigouts/0/diff", "Handle In"=w370) -> ("Handle Out"=w368:T1)  [unwired: 2 in, 1 out]
        }
        frame #18 {
          n163 = local read "MFLI-1-Settings"() -> (w374:T2)
          n164 = Unbundle By Name(w374) -> ("Offset (V)"=w371:dbl)
          n165 = call-poly "ziSetValue.vi"("Value"=w371, "Path"="sigouts/0/offset", "Handle In"=w375) -> ("Handle Out"=w373:T1)  [unwired: 2 in, 1 out]
        }
        frame #19 {
          n166 = local read "MFLI-1-Settings"() -> (w384:T2)
          n167 = Unbundle By Name(w384) -> ("Aux Out 2 Select"=w379:string)
          n168 = Unbundle By Name(w384) -> ("Aux Out 3 Select"=w377:string)
          n169 = Unbundle By Name(w384) -> ("Aux Out 1 Select"=w381:string)
          n170 = Unbundle By Name(w384) -> ("Aux Out 0 Select"=w383:string)
          n171 = flat-sequence {
            tunnel: w385 -> [w390]
            tunnel: w383 -> [w386]
            tunnel: [w389] -> w382
            tunnel: w382 -> [w392]
            tunnel: w381 -> [w395]
            tunnel: [w391] -> w380
            tunnel: w380 -> [w397]
            tunnel: w379 -> [w400]
            tunnel: [w396] -> w378
            tunnel: w378 -> [w402]
            tunnel: w377 -> [w405]
            tunnel: [w401] -> w376
            frame #0 {
              n172 = Decimal String To Number(string=w386) -> (number=w387:i32)  [unwired: 2 in, 1 out]
              n173 = call-poly "ziSetValue.vi"("Value"=w387, "Path"="auxouts/0/outputselect", "Handle In"=w390) -> ("Handle Out"=w389:T1)  [unwired: 2 in, 1 out]
            }
            frame #1 {
              n174 = Decimal String To Number(string=w395) -> (number=w394:i32)  [unwired: 2 in, 1 out]
              n175 = call-poly "ziSetValue.vi"("Value"=w394, "Path"="auxouts/1/outputselect", "Handle In"=w392) -> ("Handle Out"=w391:T1)  [unwired: 2 in, 1 out]
            }
            frame #2 {
              n176 = Decimal String To Number(string=w400) -> (number=w399:i32)  [unwired: 2 in, 1 out]
              n177 = call-poly "ziSetValue.vi"("Value"=w399, "Path"="auxouts/2/outputselect", "Handle In"=w397) -> ("Handle Out"=w396:T1)  [unwired: 2 in, 1 out]
            }
            frame #3 {
              n178 = Decimal String To Number(string=w405) -> (number=w404:i32)  [unwired: 2 in, 1 out]
              n179 = call-poly "ziSetValue.vi"("Value"=w404, "Path"="auxouts/3/outputselect", "Handle In"=w402) -> ("Handle Out"=w401:T1)  [unwired: 2 in, 1 out]
            }
          }
        }
        frame #20 {
          n180 = local read "MFLI-1-Settings"() -> (w414:T2)
          n181 = Unbundle By Name(w414) -> ("Aux Out 2 Demod Num"=w409:dbl)
          n182 = Unbundle By Name(w414) -> ("Aux Out 3 Demod Num"=w407:dbl)
          n183 = Unbundle By Name(w414) -> ("Aux Out 0 Demod Num"=w413:dbl)
          n184 = Unbundle By Name(w414) -> ("Aux Out 1 Demod Num"=w411:dbl)
          n185 = flat-sequence {
            tunnel: w415 -> [w419]
            tunnel: w413 -> [w416]
            tunnel: [w418] -> w412
            tunnel: w412 -> [w421]
            tunnel: w411 -> [w423]
            tunnel: [w420] -> w410
            tunnel: w410 -> [w425]
            tunnel: w409 -> [w427]
            tunnel: [w424] -> w408
            tunnel: w408 -> [w429]
            tunnel: w407 -> [w431]
            tunnel: [w428] -> w406
            frame #0 {
              n186 = call-poly "ziSetValue.vi"("Value"=w416, "Path"="auxouts/0/demodselect", "Handle In"=w419) -> ("Handle Out"=w418:T1)  [unwired: 2 in, 1 out]
            }
            frame #1 {
              n187 = call-poly "ziSetValue.vi"("Value"=w423, "Path"="auxouts/1/demodselect", "Handle In"=w421) -> ("Handle Out"=w420:T1)  [unwired: 2 in, 1 out]
            }
            frame #2 {
              n188 = call-poly "ziSetValue.vi"("Value"=w427, "Path"="auxouts/2/demodselect", "Handle In"=w425) -> ("Handle Out"=w424:T1)  [unwired: 2 in, 1 out]
            }
            frame #3 {
              n189 = call-poly "ziSetValue.vi"("Value"=w431, "Path"="auxouts/3/demodselect", "Handle In"=w429) -> ("Handle Out"=w428:T1)  [unwired: 2 in, 1 out]
            }
          }
        }
        frame #21 {
          n190 = local read "MFLI-1-Settings"() -> (w440:T2)
          n191 = Unbundle By Name(w440) -> ("Aux Out 0 Pre Offset"=w439:dbl)
          n192 = Unbundle By Name(w440) -> ("Aux Out 1 Pre Offset"=w437:dbl)
          n193 = Unbundle By Name(w440) -> ("Aux Out 2 Pre Offset"=w435:dbl)
          n194 = Unbundle By Name(w440) -> ("Aux Out 3 Pre Offset"=w433:dbl)
          n195 = flat-sequence {
            tunnel: w441 -> [w445]
            tunnel: w439 -> [w442]
            tunnel: [w444] -> w438
            tunnel: w438 -> [w447]
            tunnel: w437 -> [w449]
            tunnel: [w446] -> w436
            tunnel: w436 -> [w451]
            tunnel: w435 -> [w453]
            tunnel: [w450] -> w434
            tunnel: w434 -> [w455]
            tunnel: w433 -> [w457]
            tunnel: [w454] -> w432
            frame #0 {
              n196 = call-poly "ziSetValue.vi"("Value"=w442, "Path"="auxouts/0/preoffset", "Handle In"=w445) -> ("Handle Out"=w444:T1)  [unwired: 2 in, 1 out]
            }
            frame #1 {
              n197 = call-poly "ziSetValue.vi"("Value"=w449, "Path"="auxouts/1/preoffset", "Handle In"=w447) -> ("Handle Out"=w446:T1)  [unwired: 2 in, 1 out]
            }
            frame #2 {
              n198 = call-poly "ziSetValue.vi"("Value"=w453, "Path"="auxouts/2/preoffset", "Handle In"=w451) -> ("Handle Out"=w450:T1)  [unwired: 2 in, 1 out]
            }
            frame #3 {
              n199 = call-poly "ziSetValue.vi"("Value"=w457, "Path"="auxouts/3/preoffset", "Handle In"=w455) -> ("Handle Out"=w454:T1)  [unwired: 2 in, 1 out]
            }
          }
        }
        frame #22 {
          n200 = local read "MFLI-1-Settings"() -> (w466:T2)
          n201 = Unbundle By Name(w466) -> ("Aux Out 2 Scale"=w461:dbl)
          n202 = Unbundle By Name(w466) -> ("Aux Out 1 Scale"=w463:dbl)
          n203 = Unbundle By Name(w466) -> ("Aux Out 3 Scale"=w459:dbl)
          n204 = Unbundle By Name(w466) -> ("Aux Out 0 Scale"=w465:dbl)
          n205 = flat-sequence {
            tunnel: w467 -> [w471]
            tunnel: w465 -> [w468]
            tunnel: [w470] -> w464
            tunnel: w464 -> [w473]
            tunnel: w463 -> [w475]
            tunnel: [w472] -> w462
            tunnel: w462 -> [w477]
            tunnel: w461 -> [w479]
            tunnel: [w476] -> w460
            tunnel: w460 -> [w481]
            tunnel: w459 -> [w483]
            tunnel: [w480] -> w458
            frame #0 {
              n206 = call-poly "ziSetValue.vi"("Value"=w468, "Path"="auxouts/0/scale", "Handle In"=w471) -> ("Handle Out"=w470:T1)  [unwired: 2 in, 1 out]
            }
            frame #1 {
              n207 = call-poly "ziSetValue.vi"("Value"=w475, "Path"="auxouts/1/scale", "Handle In"=w473) -> ("Handle Out"=w472:T1)  [unwired: 2 in, 1 out]
            }
            frame #2 {
              n208 = call-poly "ziSetValue.vi"("Value"=w479, "Path"="auxouts/2/scale", "Handle In"=w477) -> ("Handle Out"=w476:T1)  [unwired: 2 in, 1 out]
            }
            frame #3 {
              n209 = call-poly "ziSetValue.vi"("Value"=w483, "Path"="auxouts/3/scale", "Handle In"=w481) -> ("Handle Out"=w480:T1)  [unwired: 2 in, 1 out]
            }
          }
        }
        frame #23 {
          n210 = local read "MFLI-1-Settings"() -> (w492:T2)
          n211 = Unbundle By Name(w492) -> ("Aux Out 1 Offset"=w489:dbl)
          n212 = Unbundle By Name(w492) -> ("Aux Out 3 Offset"=w485:dbl)
          n213 = Unbundle By Name(w492) -> ("Aux Out 0 Offset"=w491:dbl)
          n214 = Unbundle By Name(w492) -> ("Aux Out 2 Offset"=w487:dbl)
          n215 = flat-sequence {
            tunnel: w493 -> [w497]
            tunnel: w491 -> [w494]
            tunnel: [w496] -> w490
            tunnel: w490 -> [w499]
            tunnel: w489 -> [w501]
            tunnel: [w498] -> w488
            tunnel: w488 -> [w503]
            tunnel: w487 -> [w505]
            tunnel: [w502] -> w486
            tunnel: w486 -> [w507]
            tunnel: w485 -> [w509]
            tunnel: [w506] -> w484
            frame #0 {
              n216 = call-poly "ziSetValue.vi"("Value"=w494, "Path"="auxouts/0/offset", "Handle In"=w497) -> ("Handle Out"=w496:T1)  [unwired: 2 in, 1 out]
            }
            frame #1 {
              n217 = call-poly "ziSetValue.vi"("Value"=w501, "Path"="auxouts/0/offset", "Handle In"=w499) -> ("Handle Out"=w498:T1)  [unwired: 2 in, 1 out]
            }
            frame #2 {
              n218 = call-poly "ziSetValue.vi"("Value"=w505, "Path"="auxouts/0/offset", "Handle In"=w503) -> ("Handle Out"=w502:T1)  [unwired: 2 in, 1 out]
            }
            frame #3 {
              n219 = call-poly "ziSetValue.vi"("Value"=w509, "Path"="auxouts/0/offset", "Handle In"=w507) -> ("Handle Out"=w506:T1)  [unwired: 2 in, 1 out]
            }
          }
        }
        frame #24 {
          n220 = local read "MFLI-1-Settings"() -> (w513:T2)
          n221 = Unbundle By Name(w513) -> ("Range (V)"=w510:dbl)
          n222 = call-poly "ziSetValue.vi"("Value"=w510, "Path"="sigins/0/range", "Handle In"=w514) -> ("Handle Out"=w512:T1)  [unwired: 2 in, 1 out]
        }
      }
    }
  }
  "Handle Out" <- w2
